vi "Euler Global.vi"() -> ()   [LabVIEW 2020, in "NI_Gmath.lvlib"]
uses:
  <vilib>/gmath/NI_Gmath.lvlib
panel:
  in  "time":string="t"
  in  "X":string[](array[string])=["x1", "x2"]
  out "result":dbl[][](array[numeric]) format="%.2f"
  out "table":i32[][][](array[numeric])
  # "operator"
  # "register1"
  # "register2"
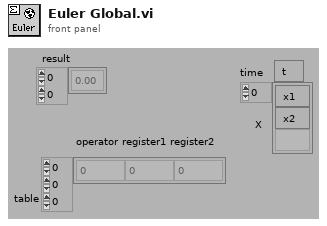
[diagram p1: front panel]
diagram:
